vi "buildTerminalName.vi"(8 "error in (no error)":errorcluster, 9 "Local Terminal Name":string, 10 "Channel Name":string, 11 "session handle":refnum<k15>) -> (0 "error IO":errorcluster, 2 "Fully Qualified Terminal Name":string, 3 "session handle 2":refnum<k15>)   [LabVIEW 2020]
doc: "This SubVI builds a fully qualified terminal name (such as \"/dev1/Engine0/StartTrigger\") based off of the device name, desired channel and desired local terminal name."
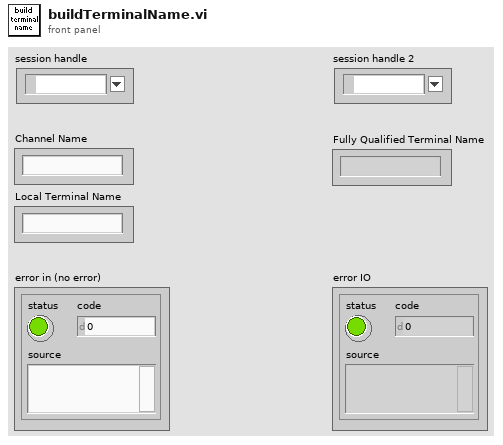
[diagram p1: front panel]
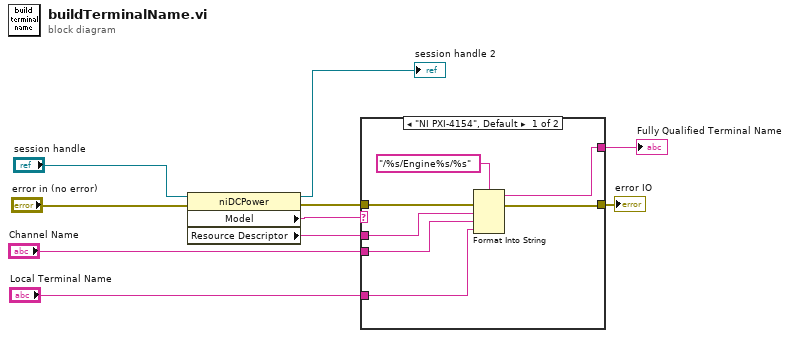
[diagram p0: block diagram]
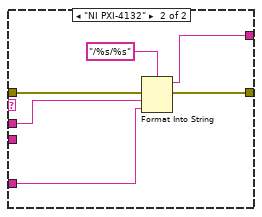
[diagram p2: hidden frame]
diagram:
  n1 = property class="niDCPower"(reference="session handle", error in="error in (no error)") -> (reference out=→"session handle 2":refnum<k15>, error out=w6:errorcluster, "Model"=w10:string, "Resource Descriptor"=w3:string)
  n2 = case shown="\"NI PXI-4154\", Default" w10 {
    tunnel: w6 -> [w17 w23]
    tunnel: [w16 w22] -> w5
    tunnel: [w15 w21] -> w4
    tunnel: w3 -> [w13 w19]
    tunnel: "Channel Name" -> [w12 _]
    tunnel: "Local Terminal Name" -> [w11 w18]
    frame "NI PXI-4154", Default {
      n3 = Format Into String(format string="/%s/Engine%s/%s", error in=w17, w13, w12, w11) -> (resulting string=w15:string, error out=w16:errorcluster)  [unwired: 1 in]
    }
    frame "NI PXI-4132" {
      n4 = Format Into String(format string="/%s/%s", error in=w23, w19, w18) -> (resulting string=w21:string, error out=w22:errorcluster)  [unwired: 1 in]
    }
  }
  "error IO" <- w5
  "Fully Qualified Terminal Name" <- w4
